vi "Find Peaks from XY.vi"(8 "width":i32(slide)=218 scale=0.0..200.0, 9 "peaks/valleys":u16(ring) items=["Peaks", "Valleys"], 10 "Y Axis":dbl[](array[numeric]), 11 "X Axis":dbl[](array[numeric])) -> (1 "Peak Index Position":dbl[](array[numeric]), 2 "Peak Magnitude":dbl[](array[numeric]), 3 "Peak X Position":dbl[](array[numeric]))   [LabVIEW 2010]
uses:
  <vilib>/measure/mamon.llb/Waveform Peak Detection for 1 Chan.vi
  <vilib>/measure/NI_MAPro.lvlib
  <vilib>/Analysis/NI_AALBase.lvlib
panel:
  out "Threshold":dbl=372.3185
  out "X-axis RSD":dbl=0.044940413014478764 format="%#_g%"
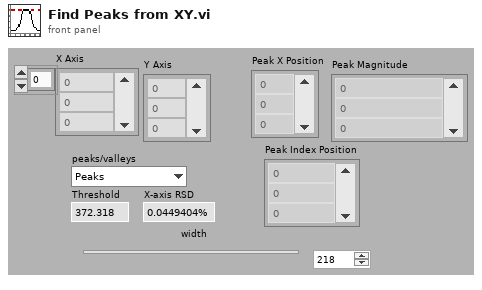
[diagram p1: front panel]
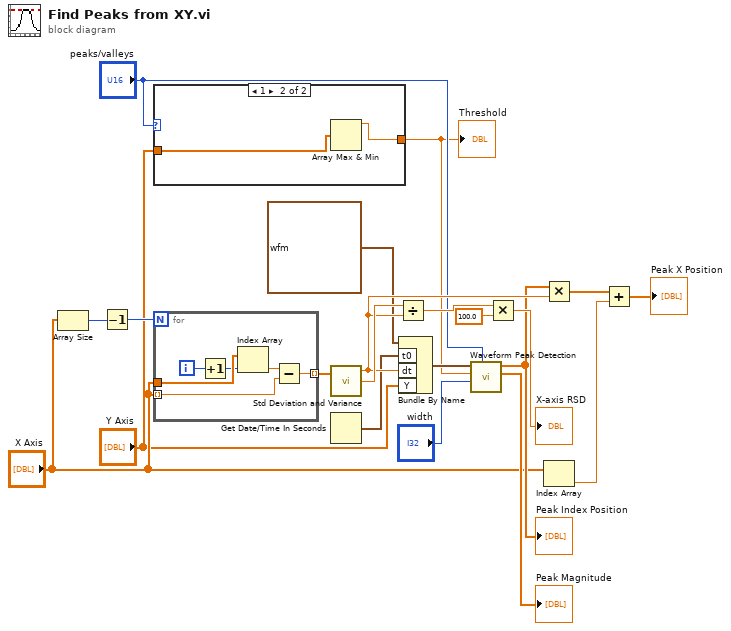
[diagram p0: block diagram]
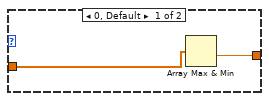
[diagram p2: hidden frame]
diagram:
  n1 = Array Size(array="X Axis") -> (size(s)=w6:i32)
  n2 = Decrement(x=w6) -> (x-1=w5:i32)
  n3 = case shown="1" "peaks/valleys" {
    tunnel: "Y Axis" -> [w23 w25]
    tunnel: [w22 w24] -> w1
    frame 0, Default {
      n4 = Array Max & Min(array=w23) -> (min value=w22:dbl)  [unwired: 3 out]
    }
    frame 1 {
      n5 = Array Max & Min(array=w25) -> (max value=w24:dbl)  [unwired: 3 out]
    }
  }
  "Threshold" <- w1
  n6 = for {
    N: w5 -> [_]
    tunnel: "X Axis" -> [w27] mode=indexing
    tunnel: "X Axis" -> [w31]
    tunnel: [w26] -> w17 mode=indexing
    i -> [w30]
    n7 = Increment(x=w30) -> (x+1=w29:i32)
    n8 = Index Array(array=w31, index=w29) -> (element=w28:dbl)
    n9 = Subtract(x=w28, y=w27) -> (x-y=w26:dbl)
  }
  n10 = call <vilib>:"Std Deviation and Variance.vi"("X"=w17) -> ("mean"=w16:dbl, "standard deviation"=w18:dbl)  [unwired: 1 in, 1 out]
  n11 = Get Date/Time In Seconds() -> (seconds since 1Jan1904=w11:timestamp)
  n12 = Divide(x=w18, y=w16) -> (x/y=w20:dbl)
  n13 = Bundle By Name(cluster=waveform(dbl) {"t0"=timestamp(0 s since 1904-01-01), "dt"=1.0, "Y"=[]} ("waveform"), "t0"=w11, "dt"=w16, "Y"="Y Axis") -> (w13:waveform(dbl))
  n14 = call-poly <vilib>:"Waveform Peak Detection.vi"("peaks/valleys"="peaks/valleys", "width"="width", "threshold"=w1, "Signal In"=w13) -> ("Amplitudes"=→"Peak Magnitude":dbl[], "Locations"=w7:dbl[])  [unwired: 3 in, 3 out]
  "Peak Index Position" <- w7
  n15 = Multiply(x=w20, y=100.0) -> (x*y=→"X-axis RSD":dbl)
  n16 = Multiply(x=w7, y=w16) -> (x*y=w15:dbl[])
  n17 = Index Array(array="X Axis") -> (element=w14:dbl)  [unwired: 1 in]
  n18 = Add(x=w15, y=w14) -> (x+y=→"Peak X Position":dbl[])
